vi "Test Convert.vi"(11 "Error in":errorcluster) -> (15 "Error out":errorcluster)   [LabVIEW 2020, in "CelsiusToFarenheitTests.lvlib"]
doc: "This VI is to validate Celsius to farenheit"
uses:
  CelsiusToFarenheitTests.lvlib
  <vilib>/SLL Drona/APIs/Stimulus/ControlValue/ValueSignalByPathString.vi
  <vilib>/SLL Drona/APIs/Assert/AssertControlValue/AlmostEqual.vi
  <vilib>/SLL Drona/APIs/Stimulus/VI/CloseVI.vi
  <vilib>/Utility/error.llb/Error Cluster From Error Code.vi
  <vilib>/ErrorRing/Error Ring.xnode
  <vilib>/SLL Drona/Drona.lvlib
  <vilib>/addons/_JKI Toolkits/Caraya/classes/Test/Test.lvclass
  <vilib>/SLL Drona/APIs/Stimulus/VI/VI.lvlib
  <vilib>/SLL Drona/APIs/Stimulus/ControlValue/ControlValue.lvlib
  <vilib>/SLL Drona/APIs/Assert/AssertControlValue/AssertControlValue.lvlib
  <vilib>/Wiresmith Technology/G CLI/CLI Class/CLI.lvclass
panel:
  # "CELSIUS TO FAHRENHEIT TEST"
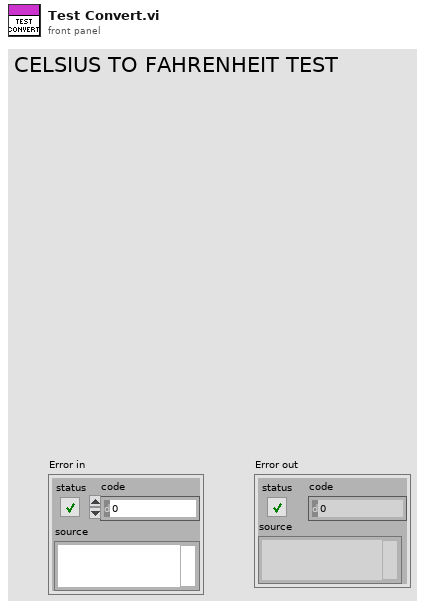
[diagram p1: front panel]
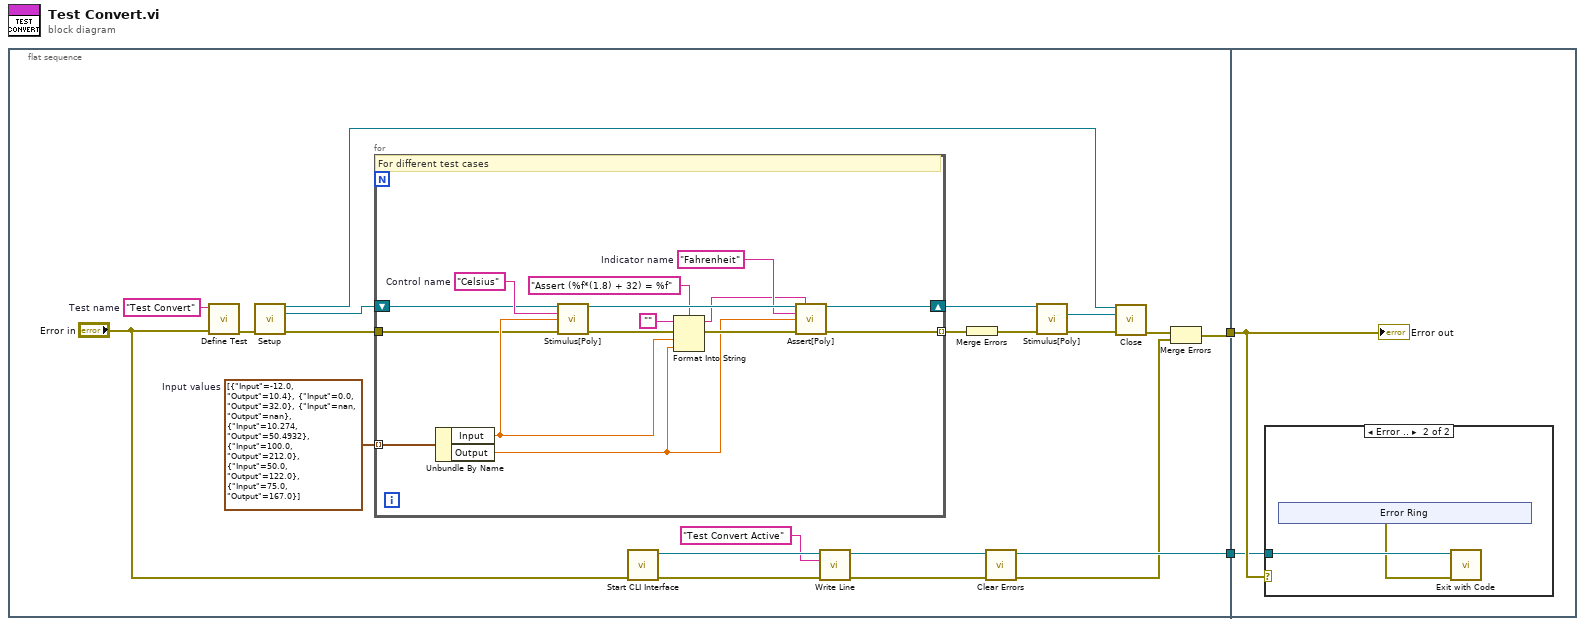
[diagram p0: block diagram]
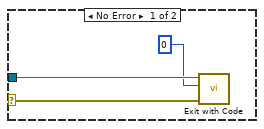
[diagram p2: hidden frame]
diagram:
  n1 = flat-sequence {
    tunnel: [w7] -> w2
    tunnel: [w9] -> w1
    tunnel: w2 -> [w39]
    tunnel: w1 -> [w38]
    frame #0 {
      w14 = "Test Convert"  # Test name
      w22 = cluster{"Input":dbl, "Output":dbl}[] [{"Input"=-12.0, "Output"=10.4}, {"Input"=0.0, "Output"=32.0}, {"Input"=nan, "Output"=nan}, {"Input"=10.274, "Output"=50.4932}, {"Input"=100.0, "Output"=212.0}, {"Input"=50.0, "Output"=122.0}, {"Input"=75.0, "Output"=167.0}]  # Input values
      n2 = call <vilib>:"Define Test.vi"("error in (no error)"="Error in", "Label (VI Title)"=w14) -> ("error out"=w6:errorcluster)  [unwired: 9 in]
      n3 = call <vilib>:"Setup.vi"("error in"=w6) -> ("Application Ref"=w20:refnum<vi>, "VI Reference Out"=w21:refnum<vi>, "error out"=w15:errorcluster)  [unwired: 12 in]
      n4 = for {
        tunnel: w22 -> [w37] mode=indexing
        shift-right: [w27] -> w19
        shift-left: w21 -> [w35]
        tunnel: w15 -> [w24]
        tunnel: [w23] -> w17 mode=indexing
        w28 = "Fahrenheit"  # Indicator name
        w36 = "Celsius"  # Control name
        # "For different test cases"
        n5 = Unbundle By Name(w37) -> ("Input"=w25:dbl, "Output"=w29:dbl)
        n6 = call-poly <vilib>:"Stimulus[Poly].vi"("VI Reference In"=w35, "Control Path"=w36, "Value (Signaling)"=w25, "error in"=w24) -> ("VI Reference Out"=w31:refnum<vi>, "error out"=w33:errorcluster)  [unwired: 10 in]
        n7 = Format Into String(format string="Assert (%f*(1.8) + 32) = %f", initial string="", error in=w33, w25, w29) -> (resulting string=w26:string, error out=w32:errorcluster)
        n8 = call-poly <vilib>:"Assert[Poly].vi"("VI Reference In"=w31, "Test Label"=w26, "Control Path"=w28, "Control Value"=w29, "Error In"=w32) -> ("VI Reference Out"=w27:refnum<vi>, "Error Out"=w23:errorcluster)  [unwired: 9 in]
      }
      n9 = call <vilib>:"Start CLI Interface.vi"("error in (no error)"="Error in") -> ("error out"=w12:errorcluster, "CLI out"=w11:refnum<class "CLI.lvclass">)  [unwired: 7 in, 2 out]
      n10 = call <vilib>:"Write Line.vi"("error in (no error)"=w12, "Text to Write"="Test Convert Active", "CLI in"=w11) -> ("error out"=w4:errorcluster, "CLI out"=w9:refnum<class "CLI.lvclass">)  [unwired: 7 in]
      n11 = Merge Errors(w17) -> (w13:errorcluster)
      n12 = call <vilib>:"Clear Errors.vi"("error in (no error)"=w4) -> ("error out"=w3:errorcluster)  [unwired: 5 in, 1 out]
      n13 = call-poly <vilib>:"Stimulus[Poly].vi"("VI Reference In"=w19, "error in"=w13) -> ("VI Reference Out"=w18:refnum<vi>, "error out"=w16:errorcluster)  [unwired: 12 in]
      n14 = call <vilib>:"Close.vi"("Application Ref"=w20, "VI Reference"=w18, "error in"=w16) -> ("error out"=w8:errorcluster)  [unwired: 12 in]
      n15 = Merge Errors(w8, w3) -> (w7:errorcluster)
    }
    frame #1 {
      n16 = case shown="Error .." w39 {
        selector: w39 -> [w40 _]
        tunnel: w38 -> [w42 w44]
        frame No Error {
          n17 = call <vilib>:"Exit with Code.vi"("error in (no error)"=w40, "Exit Code (0)"=0, "CLI in"=w42) -> ()  [unwired: 8 in, 1 out]
        }
        frame Error {
          n18 = xnode "Error Ring"() -> ("error out"=w43:errorcluster)
          n19 = call <vilib>:"Exit with Code.vi"("error in (no error)"=w43, "CLI in"=w44) -> ()  [unwired: 9 in, 1 out]
        }
      }
      "Error out" <- w39
    }
  }
